vi "Scratch Module Selection.vi"(8 "error in (no error)":errorcluster, 11 "Data Cluster":T1) -> (0 "error out":errorcluster)   [LabVIEW 2025]
uses:
  controls/LAB-IQ UI Data.ctl
  Traction Loop/Traction Receipe Enum.ctl
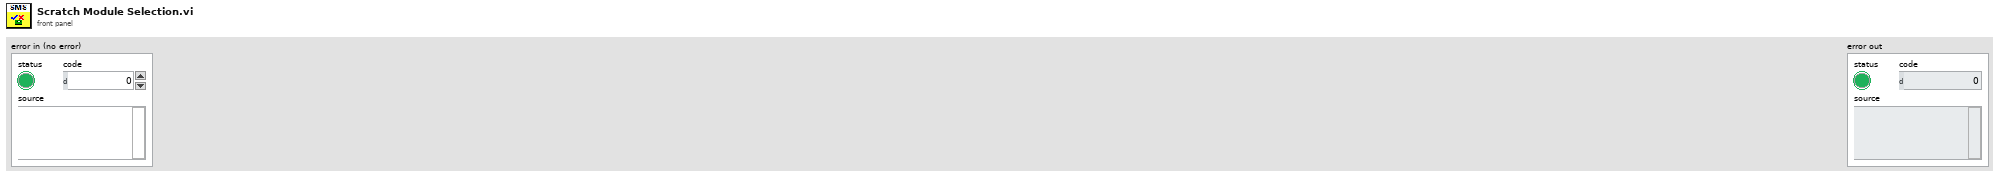
[diagram p1: front panel]
types:
  T1 = typedef "LAB-IQ UI Data.ctl" = cluster{"Main Home Screen":cluster{"GUI":refnum<vi>, "Platform Settings":refnum<vi>, "Configure":refnum<vi>, "Home":refnum<vi>, "EXIT":refnum<vi>, "service 2":refnum<vi>, "MainPage":refnum<vi>, "Analysis":refnum<vi>}, "Platform Settings":cluster{"mm/s  Surge":refnum<vi>, "Update Surge Speed":refnum<vi>, "Drive Error":refnum<vi>, "Disable Axis Jog Soft Limits":refnum<vi>, "mm/s  Sway":refnum<vi>, "Sway and Surge COM Status":refnum<vi>, "Heave COM Status":refnum<vi>, "Enable Platform":refnum<vi>, "Surge Forward Main":refnum<vi>, "Sway Right Main":refnum<vi>, "Sway Left Main":refnum<vi>, "Heave Down Main":refnum<vi>, "Heave Up main":refnum<vi>, "Update Sway Speed":refnum<vi>, "Update Heave Speed":refnum<vi>, "mm/s Heave":refnum<vi>, "mm/sec":refnum<vi>, "mm":refnum<vi>, "Surge Backward Main":refnum<vi>}, "Analysis Screen":cluster{"Analysis Home":refnum<vi>, "Surface Analysis":refnum<vi>, "Imaging":refnum<vi>, "Image Analysis":refnum<vi>, "Post Analysis":refnum<vi>}, "Config Screen":cluster{"Select Load Head":refnum<vi>, "Notes :":refnum<vi>, "FILE":refnum<vi>, "Sample ID :":refnum<vi>, "Operator ID :":refnum<vi>, "Operator Name :":refnum<vi>, "Auto":refnum<vi>}, "Motion Module":cluster{"zNL":refnum<vi>, "NL disp":refnum<vi>, "Rotary Tab":refnum<vi>, "Motion Direction:  3":refnum<vi>, "E.Velocity 2":refnum<vi>, "e.v/ssr 2":refnum<vi>, "Enter Fixed E.Velocity 2":refnum<vi>, "Enter Final SRR 2":refnum<vi>, "Enter initial SRR 2":refnum<vi>, "Enter Fixed SRR 2":refnum<vi>, "Enter the Final E.Velocity (m/s) 2":refnum<vi>, "Enter initial E.Velocity (m/s) 2":refnum<vi>, "Final Speed (RPM) 3":refnum<vi>, "Initial Speed (RPM) 2":refnum<vi>, "Enter the Final Velocity (m/s) 3":refnum<vi>, "Enter initial Velocity (m/s)  3":refnum<vi>, "Ramp Up 2":refnum<vi>, "TEST SELECTION":refnum<vi>, "SPEED SELECTION : ":refnum<vi>, "Angular Oscillation Set":refnum<vi>, "Traction":refnum<vi>, "Step Speed":refnum<vi>, "StepTable For Load-Speed":refnum<vi>, "StepTable For Speed":refnum<vi>, "Surge Forward MM":refnum<vi>, "Surge Backward MM":refnum<vi>, "M3 Image":refnum<vi>, "String 39":refnum<vi>, "Sway Left MM":refnum<vi>, "Sway Right MM":refnum<vi>, "Disable Axis Jog Soft Limits":refnum<vi>, "mm":refnum<vi>, "Heave Down MM":refnum<vi>, "Heave Up MM":refnum<vi>, "Wear Track Diameter (mm)":refnum<vi>, "Set WTD":refnum<vi>, "HomeScratch":refnum<vi>, "HomeRot":refnum<vi>, "PlaceModule":refnum<vi>, "Enter the Angle (Deg)":refnum<vi>, "Enter the Frequency (Hz)":refnum<vi>, "Motion Mode:":refnum<vi>, "LR Sway":refnum<vi>, "Rot Hor":refnum<vi>, "Scratch":refnum<vi>, "LR Cam":refnum<vi>, "MMBack":refnum<vi>, "MMNext":refnum<vi>, "Rot Ver":refnum<vi>, "Rotary Module Selection":refnum<vi>, "calculate rotary":refnum<vi>, "SPEED SELECTION : rotary":refnum<vi>, "Import 2":refnum<vi>, "Save 2":refnum<vi>, "File Path :  2":refnum<vi>, "String 45":refnum<vi>, "StepTable For Speed 3":refnum<vi>, "Enter the Speed(mm/sec)":refnum<vi>, "Enter the Speed(RPM)":refnum<vi>, "Enter Scratch Speed (mm/s):":refnum<vi>, "SwaySpeed Set":refnum<vi>, "Scartch Offset":refnum<vi>, "Motion type:":refnum<vi>, "HomeScratch 2":refnum<vi>, "Enter Scratch length (mm):":refnum<vi>, "Wear Track Diameter":refnum<vi>, "Rotary Speed Exced":refnum<vi>, "Scratch Mode":refnum<vi>, "No of Scratch":refnum<vi>}, "Environmental control":cluster{"Humidity  Status  3":refnum<vi>, "Low Temp  Status  2":refnum<vi>, "TK4 status 2":refnum<vi>, "Stage Temperature":refnum<vi>, "Sample Temperature":refnum<vi>, "Humidity (Amb)":refnum<vi>, "Clear List":refnum<vi>, "Add to list":refnum<vi>, "Wear":refnum<vi>, "Vibration":refnum<vi>, "Humidity (Chamber)":refnum<vi>, "Temperature (Chamber)":refnum<vi>, "ECR ":refnum<vi>, "Temperature (Amb)":refnum<vi>, "Microphone":refnum<vi>, "Acoustic Emission 3":refnum<vi>, "SNext":refnum<vi>, "APBack":refnum<vi>, "Enter the Temperature (°C):":refnum<vi>, "Enter the Stage \nTemperature (°C):":refnum<vi>, "Enter the Humidity (%Rh):":refnum<vi>, "Low Temp":refnum<vi>, "High Temp":refnum<vi>, "Humidity":refnum<vi>, "Sensors Picked":refnum<vi>}, "About Screen":cluster{"Password":refnum<vi>, "Home Service":refnum<vi>, "Advanced Setting":refnum<vi>, "About Tab":refnum<vi>, "ECR Port:":refnum<vi>, "Ramp Port:":refnum<vi>, "Installation/Replacement completed":refnum<vi>, "Loahead":refnum<vi>, "Heave and Surge COM Port:":refnum<vi>, "Sway COM Port:":refnum<vi>, "Temp Modbus:":refnum<vi>, "Humidity Port:":refnum<vi>, "Edit Gain Constants":refnum<vi>, "Save Gain Constants":refnum<vi>}, "Main Screen":cluster{"Main Screen Tab":refnum<vi>, "Angle and Frequency":refnum<vi>, "Stroke (mm)":refnum<vi>, "Angle (Deg)":refnum<vi>, "Main Speed Tab":refnum<vi>, "MTM MOTOR DISPLAY":refnum<vi>, "Disc Speed (m/sec)":refnum<vi>, "Ball Speed (m/sec)":refnum<vi>, "Disc Speed (RPM)":refnum<vi>, "Ball Speed (RPM)":refnum<vi>, "SPEED TAB":refnum<vi>, "Speed (m/sec)":refnum<vi>, "Set Speed (m/sec)":refnum<vi>, "Speed (RPM)":refnum<vi>, "Set Speed":refnum<vi>, "Time Tab":refnum<vi>, "Time ( HH:MM:SS ) 2":refnum<vi>, "Test Duration":refnum<vi>, "Test Duration 4":refnum<vi>, "TEST CYCLE":refnum<vi>, "TOTAL CYCLES":refnum<vi>, "Set Load (N)":refnum<vi>, "Temp Tabs":refnum<vi>, "Heater":refnum<vi>, "TK4 status":refnum<vi>, "ChamberTemp":refnum<vi>, "SetTmp":refnum<vi>, "Controller  Status":refnum<vi>, "ChamberTemp 2":refnum<vi>, "SetTmp 2":refnum<vi>, "Controller  Status 2":refnum<vi>, "ChamberTemp 3":refnum<vi>, "SetTmp 3":refnum<vi>, "Cooling":refnum<vi>, "Load Communication":refnum<vi>, "Ambient \nTemperature":refnum<vi>, "HumCOMStatus":refnum<vi>, "Ambient\n Humidity":refnum<vi>, "Freq (Hz)":refnum<vi>, "Load En":refnum<vi>, "NLt":refnum<vi>, "zNL 2":refnum<vi>, "Humidity On":refnum<vi>, "humidity disp":refnum<vi>, "Set Humidity":refnum<vi>, "NL disp 2":refnum<vi>, "Humidity On 2":refnum<vi>, "humidity disp 2":refnum<vi>, "Set Humidity 2":refnum<vi>, "NL disp 3":refnum<vi>, "AppLoadSeq scratch":refnum<vi>, "Stop Scratch":refnum<vi>, "ClrLog":refnum<vi>, "Trip Log":refnum<vi>, "STOP":refnum<vi>, "Start Test":refnum<vi>, "Test status":refnum<vi>, "AR Led":refnum<vi>, "Data":refnum<vi>, "Health":refnum<vi>, "Sway COM Status":refnum<vi>, "Heave COM Status":refnum<vi>, "Grp Tab":refnum<vi>, "Sub Graph":refnum<vi>, "SD (mm)":refnum<vi>, "Siliding distance Reset Graph":refnum<vi>, "SDGp":refnum<vi>, "Humidity Reset Graph":refnum<vi>, "HumrGp":refnum<vi>, "Acoustic Emission (mV)":refnum<vi>, "Aqucostic Reset Graph":refnum<vi>, "gACQUOS":refnum<vi>, "ECR RESET":refnum<vi>, "ECR":refnum<vi>, "Temperature Reset":refnum<vi>, "Acoustic Emission (mV) 2":refnum<vi>, "Aqucostic Reset Graph 2":refnum<vi>, "gACQUOS 2":refnum<vi>, "ECR RESET 2":refnum<vi>, "ECR 2":refnum<vi>, "Temperature Reset 2":refnum<vi>, "Temperature (deg c)":refnum<vi>, "Speed Reset Graph":refnum<vi>, "Speed Tab":refnum<vi>, "MTM DISC  SPEED":refnum<vi>, "MTM BALL SPEED":refnum<vi>, "speed mm/sec":refnum<vi>, "Hymidity":refnum<vi>, "Humidity Disable trip":refnum<vi>, "CoF Trip  2":refnum<vi>, "Depth Trip":refnum<vi>, "Weart Deapth":refnum<vi>, "Depth Reset Graph":refnum<vi>, "Weart":refnum<vi>, "Depthz":refnum<vi>, "Depth (µm)":refnum<vi>, "WearGp":refnum<vi>, "NL Trip 2":refnum<vi>, "Load pid":refnum<vi>, "Load Disable Trip":refnum<vi>, "Load Reset Graph":refnum<vi>, "NL Display 4":refnum<vi>, "Main Chart 3":refnum<vi>, "BACK":refnum<vi>, "Depth Trip 2":refnum<vi>, "COF TRIP ":refnum<vi>, "Friction Force (N)":refnum<vi>, "FF Reset Graph":refnum<vi>, "FF Disable Trip":refnum<vi>, "FF TRIP":refnum<vi>, "COF Disable Trip":refnum<vi>, "COF Reset Graph":refnum<vi>, "Start Test Temp":refnum<vi>, "zFF":refnum<vi>, "Friction Force (N) Graph":refnum<vi>, "Coefficient of Friction":refnum<vi>, "Scratch Start Test":refnum<vi>, "FF Tab":refnum<vi>, "Cyclic Friction Force (N)":refnum<vi>, "CZ FF":refnum<vi>, "Cyclic Friction Force (N) Graph":refnum<vi>, "Cyclic Coefficient of Friction":refnum<vi>, "Cyclic FF TRIP":refnum<vi>, "Cyclic FF Disable Trip":refnum<vi>, "cyclic COF Disable Trip":refnum<vi>, "cyclic COF TRIP":refnum<vi>, "cyclic COF Reset Graph":refnum<vi>, "Cyclic FF Reset Graph":refnum<vi>, "Test Trip":refnum<vi>, "Multi Scratch Pass":refnum<vi>, "Scratch Start Recording":refnum<vi>}, "Loading":cluster{"Indentation":refnum<vi>, "Reference Sample":refnum<vi>, "Load Cell Communication Slide":refnum<vi>, "com 3":refnum<vi>, "com":refnum<vi>, "DecaForce COM Status":refnum<vi>, "Update":refnum<vi>, "Clear 3":refnum<vi>, "seq":refnum<vi>, "Stribeck table":refnum<vi>, "Stribeck Table  For loading":refnum<vi>, "Loading Mode":refnum<vi>, "Enter the Final Load (N)":refnum<vi>, "Enter the CoF Trip":refnum<vi>, "Enter the Friction Force Trip":refnum<vi>, "Enter the Normal load Trip":refnum<vi>, "Enter the Load  (N)":refnum<vi>, "KiloForce":refnum<vi>, "DecaForce ":refnum<vi>, "MicroForce":refnum<vi>, "LHBack":refnum<vi>, "LHNext":refnum<vi>, "Enter the Loading Rate (N/min)":refnum<vi>, "Message":refnum<vi>, "Warning 2":refnum<vi>, "SSP 0.75":refnum<vi>, "SSP 0.5":refnum<vi>, "SSP 0.3":refnum<vi>, "Warning":refnum<vi>, "gui GIF":refnum<vi>, "Communication is established":refnum<vi>, "AppLoad 4":refnum<vi>, "Multipoint":refnum<vi>, "Load Selection":refnum<vi>}, "PID":cluster{"Ramp MulFac":refnum<vi>, "pulses LoadDiffRamp(2..10)":refnum<vi>, "PulseControlRamp(diff<=3N)":refnum<vi>, "SetLoadDeadband(%) Load(0-10N)":refnum<vi>, "PID gains out delay (microForce)":refnum<vi>, "Ramp":refnum<vi>, "Gain 2":refnum<vi>, "pulses LoadDiff(2..10)":refnum<vi>, "pulses LoadDiff(11..50)":refnum<vi>, "PulseControl(diff<=3N)":refnum<vi>, "SetLoadDeadband(%)  2":refnum<vi>, "Dummy Run":refnum<vi>, "Vertical load (N)":refnum<vi>, "AutoTune":refnum<vi>, "Offset 3 ":refnum<vi>, "apply load":refnum<vi>, "Offset  3":refnum<vi>, "apply load 2":refnum<vi>, "Enter ByPass Load":refnum<vi>, "reinit 3":refnum<vi>, "output range delay":refnum<vi>, "PID gains out delay":refnum<vi>, "Bypass Load":refnum<vi>, "pulsesSent":refnum<vi>, "pulses ":refnum<vi>, "actpid":refnum<vi>, "gFF Rot":refnum<vi>, "pulses LoadDiff(21..1000)":refnum<vi>, "Delay":refnum<vi>, "deadband":refnum<vi>}, "Config Parameters":cluster{"Tab Control 3":refnum<vi>, "Tab Control 19":refnum<vi>, "SAMPLES":refnum<vi>, "Re-initilaize":refnum<vi>, "Filter ON/OFF":refnum<vi>, "TracHomeSurgeOffsetCounts 10MM":refnum<vi>, "TracHomeSwayOffsetCounts 10MM":refnum<vi>, "Acoustic Emission:":refnum<vi>, "Apply Filter (FF)":refnum<vi>, "Filter% 2":refnum<vi>, "Apply Filter (Load)":refnum<vi>, "Filter% ":refnum<vi>, "Sway distance (mm)":refnum<vi>, "Surge distance (mm)":refnum<vi>, "DataSavingLoopDelay(ms)":refnum<vi>, "SAVE 2":refnum<vi>, "Enter Distance":refnum<vi>, "Sway Counts:":refnum<vi>, "Distance (mm): 3":refnum<vi>, "Surge Counts:":refnum<vi>, "Distance (mm): 2":refnum<vi>, "Distance (mm):":refnum<vi>, "Heave Counts:":refnum<vi>, "LRMHomeSurgeOffsetCounts":refnum<vi>, "LRMHomeSwayOffsetCounts":refnum<vi>, "TracHomeSurgeOffsetCounts 20MM":refnum<vi>, "TracHomeSwayOffsetCounts 20MM":refnum<vi>, "RotHomeSwayOffsetCounts":refnum<vi>, "RotHomeSurgeOffsetCounts":refnum<vi>, "Heave distance":refnum<vi>, "Zmm":refnum<vi>, "Heave Pulses/mm":refnum<vi>, "Surge Pulses/mm":refnum<vi>, "Sway Pulses/mm":refnum<vi>, "Heave Pitch":refnum<vi>, "Surge Pitch":refnum<vi>, "Sway Pitch":refnum<vi>, "Heave PPR":refnum<vi>, "Surge PPR":refnum<vi>, "Sway PPR":refnum<vi>, "Tab Control 5":refnum<vi>, "Tab Control 14":refnum<vi>, "Tab Control 26":refnum<vi>, "AE":refnum<vi>, "Heave Loop Delay":refnum<vi>, "Heave PID Speed":refnum<vi>, "Surge Jog Speed":refnum<vi>, "Heave Jog Speed":refnum<vi>, "Sway Loop Delay":refnum<vi>, "Sway PID Speed":refnum<vi>, "Sway Jog Speed":refnum<vi>, "DEPTH TRIP VALUE":refnum<vi>, "LOAD TRIP VALUE":refnum<vi>, "DEPTH TRIP   ENABLE":refnum<vi>, "LOAD TRIP  ENABLE":refnum<vi>, "CYCLIC FF TRIP VALUE":refnum<vi>, "FF TRIP VALUE":refnum<vi>, "CYCLIC CoF TRIP VALUE":refnum<vi>, "COF TRIP VALUE":refnum<vi>, "CYCLIC COF TRIP  ENABLE":refnum<vi>, "CYCLIC FF TRIP  ENABLE":refnum<vi>, "FF TRIP  ENABLE":refnum<vi>, "COF TRIP  ENABLE":refnum<vi>, "JOG TRIP LOAD VALUE (N)":refnum<vi>}, "Loading Com Port":cluster{"ClearAll":refnum<vi>, "Mz(Nm)":refnum<vi>, "My(Nm)":refnum<vi>, "Mx(Nm)":refnum<vi>, "Save Dwell":refnum<vi>, "Mx ":refnum<vi>, "My ":refnum<vi>, "Mz":refnum<vi>, "Fx(N)":refnum<vi>, "Fy(N)":refnum<vi>, "Fz(N)":refnum<vi>, "ZeroAll":refnum<vi>, "Acq Delay (ms)":refnum<vi>, "Burst Delay (ms)":refnum<vi>, "model":refnum<vi>, "SN":refnum<vi>, "FFx(N)":refnum<vi>, "Sensor IP":refnum<vi>, "Port":refnum<vi>, "FFy(N)":refnum<vi>, "Load(N)":refnum<vi>, "delete Handle":refnum<vi>, "Create Handle":refnum<vi>, "ft_data":refnum<vi>, "ft_range":refnum<vi>, "ft_data 2":refnum<vi>, "stop 6":refnum<vi>, "running_flag":refnum<vi>, "ft_udp_handle":refnum<vi>, "get-data-return":refnum<vi>, "get-range-return":refnum<vi>, "zero-return":refnum<vi>, "filter-return":refnum<vi>, "initial-return":refnum<vi>, "deleteHandle-result":refnum<vi>, "Load Cell Temp":refnum<vi>}, "Heave AND Surge":cluster{"SURGE POSE":refnum<vi>, "error out Read":refnum<vi>, "HEAVE POSE":refnum<vi>, "State":refnum<vi>, "Homed":refnum<vi>, "Sequence ID":refnum<vi>, "error out Write":refnum<vi>, "faultCode":refnum<vi>, "Ack ID":refnum<vi>, "SPEED":refnum<vi>, "Distance":refnum<vi>, "Mode Command":refnum<vi>, "Heave and Surge Read":refnum<vi>, "Read Heave Temp":refnum<vi>, "Spare 15":refnum<vi>, "Spare 14":refnum<vi>, "Spare 13":refnum<vi>, "Spare 12":refnum<vi>, "Spare 11":refnum<vi>, "Spare 10":refnum<vi>, "Spare 9":refnum<vi>, "Spare 8":refnum<vi>, "Spare 7":refnum<vi>, "Spare 6":refnum<vi>, "Spare 5":refnum<vi>, "Spare 4":refnum<vi>, "Spare 2":refnum<vi>, "Spare 1":refnum<vi>, "Node Id":refnum<vi>, "Spare 3":refnum<vi>, "SPARE 4":refnum<vi>, "SPARE 3":refnum<vi>, "SPARE 2":refnum<vi>, "SPARE 1":refnum<vi>, "fwMajor":refnum<vi>, "fwMinor":refnum<vi>, "Manual Write":refnum<vi>, "Heave and Surge Write":refnum<vi>, "SPARE 5":refnum<vi>, "Reserved ":refnum<vi>, "SPARE 8":refnum<vi>, "SPARE 6":refnum<vi>, "SPARE 7":refnum<vi>, "SPARE 17":refnum<vi>, "SPARE 16":refnum<vi>, "SPARE 15":refnum<vi>, "SPARE 14":refnum<vi>, "SPARE 13":refnum<vi>, "SPARE 12":refnum<vi>, "SPARE 11":refnum<vi>, "SPARE 10":refnum<vi>, "SPARE 9":refnum<vi>, "System UPTIME":refnum<vi>, "Missed Packets":refnum<vi>, "faultCode Surge Right":refnum<vi>, "faultCode Surge Left":refnum<vi>, "faultCode Heave":refnum<vi>}, "New PID LOGIC":cluster{"Fine Tune Zone":refnum<vi>, "PID SDelay":refnum<vi>, "Max_pos_limit":refnum<vi>, "Min_pos_limit":refnum<vi>, "i_limit":refnum<vi>, "pct_scale":refnum<vi>, "Deadband":refnum<vi>, "Kd":refnum<vi>, "Ki":refnum<vi>, "Kp":refnum<vi>, "Current Position":refnum<vi>, "Set Load":refnum<vi>, "Current Load":refnum<vi>, "Pulse delta":refnum<vi>, "Init Step":refnum<vi>, "Max Step Linit":refnum<vi>, "min_deadband_floor":refnum<vi>, "dynamic_spindle_noise_scalar":refnum<vi>, "min_finetune_floor":refnum<vi>, "filter_alpha":refnum<vi>}, "SWAY ":cluster{"fwMajor":refnum<vi>, "Homed":refnum<vi>, "Rotary POSE":refnum<vi>, "State":refnum<vi>, "SWAY POSE":refnum<vi>, "Ack ID":refnum<vi>, "faultCode":refnum<vi>, "Node Id":refnum<vi>, "fwMinor":refnum<vi>, "Spare 6":refnum<vi>, "Spare 5":refnum<vi>, "Spare 4":refnum<vi>, "Spare 3":refnum<vi>, "Spare 2":refnum<vi>, "Spare 1":refnum<vi>, "Spare 7":refnum<vi>, "SPARE  5":refnum<vi>, "error out Write  SWAY ":refnum<vi>, "error out Read SWAY ":refnum<vi>, "Manual Write SWAY ":refnum<vi>, "SWAY WRITE":refnum<vi>, "SPARE  4":refnum<vi>, "SPARE  3":refnum<vi>, "SPARE 2":refnum<vi>, "SPARE 1":refnum<vi>, "Spare 15":refnum<vi>, "Spare 14":refnum<vi>, "Spare 13":refnum<vi>, "Spare 12":refnum<vi>, "Spare 11":refnum<vi>, "Spare 9":refnum<vi>, "Spare 8":refnum<vi>, "SPEED":refnum<vi>, "Distance":refnum<vi>, "Mode Command":refnum<vi>, "Sequence ID":refnum<vi>, "SWAY READ":refnum<vi>, "Spare 10":refnum<vi>, "Read SWAY Temp":refnum<vi>, "faultCode Sway ":refnum<vi>, "Missed Packets":refnum<vi>, "System UPTIME sway":refnum<vi>, "SPARE 6":refnum<vi>, "SPARE 7":refnum<vi>, "SPARE 9":refnum<vi>, "SPARE 11":refnum<vi>, "SPARE 10":refnum<vi>, "SPARE 8":refnum<vi>, "SPARE 13":refnum<vi>, "SPARE 12":refnum<vi>, "SPARE 17":refnum<vi>, "SPARE 16":refnum<vi>, "SPARE 15":refnum<vi>, "SPARE 14":refnum<vi>, "Reserved":refnum<vi>, "faultCode Rotary":refnum<vi>}, "Analysis Screen":cluster{"Analysis Home":refnum<vi>, "Refresh 2":refnum<vi>, "MEAN 4":refnum<vi>, "SD 4":refnum<vi>, "VARIANCE 4":refnum<vi>, "MEAN  3":refnum<vi>, "SD  3":refnum<vi>, "VARIANCE  3":refnum<vi>, "MEAN 2":refnum<vi>, "SD  2":refnum<vi>, "VARIANCE 2":refnum<vi>, "MEAN":refnum<vi>, "SD":refnum<vi>, "VARIANCE":refnum<vi>, "File 4 Discription":refnum<vi>, "OPEN 4":refnum<vi>, "File Name 4":refnum<vi>, "OPEN 3":refnum<vi>, "File 3 Discription":refnum<vi>, "File Name 3":refnum<vi>, "Y-AXIS":refnum<vi>, "X-AXIS":refnum<vi>, "XY Graph":refnum<vi>, "File Name 2":refnum<vi>, "File Name 1":refnum<vi>, "OPEN 2":refnum<vi>, "OPEN 1":refnum<vi>, "File 1 Discription ":refnum<vi>, "File 2 Discription":refnum<vi>, "Export":refnum<vi>, "File Format":refnum<vi>}, "Traction":cluster{"faultCode Traction 2":refnum<vi>, "faultCode Traction 1":refnum<vi>, "Missed Packets":refnum<vi>, "System UPTIME Traction":refnum<vi>, "SPARE 17":refnum<vi>, "SPARE 16":refnum<vi>, "SPARE 15":refnum<vi>, "SPARE 14":refnum<vi>, "SPARE 13":refnum<vi>, "SPARE 12":refnum<vi>, "SPARE 11":refnum<vi>, "SPARE 10":refnum<vi>, "SPARE 9":refnum<vi>, "SPARE 8":refnum<vi>, "SPARE 7":refnum<vi>, "SPARE 6":refnum<vi>, "Reserved":refnum<vi>, "SPARE  5":refnum<vi>, "Manual Write TRACTION":refnum<vi>, "TRACTION WRITE":refnum<vi>, "SPARE  4":refnum<vi>, "SPARE  3":refnum<vi>, "SPARE 2":refnum<vi>, "SPARE 1":refnum<vi>, "Spare 7":refnum<vi>, "Spare 6":refnum<vi>, "Spare 5":refnum<vi>, "Spare 4":refnum<vi>, "Spare 2":refnum<vi>, "Spare 1":refnum<vi>, "Node Id":refnum<vi>, "Read TRACTION Temp":refnum<vi>, "fwMinor":refnum<vi>, "fwMajor":refnum<vi>, "faultCode":refnum<vi>, "TRACTION POSE":refnum<vi>, "TRACTION POSE 2":refnum<vi>, "Homed":refnum<vi>, "State":refnum<vi>, "Ack ID":refnum<vi>, "SPEED":refnum<vi>, "Distance":refnum<vi>, "Mode Command":refnum<vi>, "Sequence ID":refnum<vi>, "error out Read TRACTION":refnum<vi>, "error out Write  TRACTION":refnum<vi>, "TRACTION READ":refnum<vi>, "Spare 3":refnum<vi>}, "Traction reciepe":cluster{"SRR Sweep Range (%) Stribeck":refnum<vi>, "Traction Receipe":refnum<vi>, "Total Execution Time":refnum<vi>, "Total Steps":refnum<vi>, "Duration / Step (s)  Stribeck":refnum<vi>, "STRIBECK Fixed SRR List (%)":refnum<vi>, "Duration / Step (s) Traction":refnum<vi>, "SRR Sweep Range (%) traction":refnum<vi>, "Rolling Speed (mm/s)":refnum<vi>, "Temperature Stages (°C)":refnum<vi>, "Ball Load (N)":refnum<vi>, "Lubricant Name":refnum<vi>, "Profile File Name":refnum<vi>, "SET entrainment Velocity":refnum<vi>, "Test Array Size":refnum<vi>, "SRR INDEX [ STRIBECK]":refnum<vi>, "Stribeck Size":refnum<vi>, "SET SRR":refnum<vi>, "ELAPSED TIMER ":refnum<vi>, "BALL SET RPM":refnum<vi>, "DISC SET RPM":refnum<vi>, "SET LOAD":refnum<vi>, "TEMPERATURE READ":refnum<vi>, "SET TEMPERATURE":refnum<vi>, "Traction Size":refnum<vi>, "DISC SPEED (rpm)":refnum<vi>, "BALL SPEED (rpm)":refnum<vi>, "BALL WEAR TRACK":refnum<vi>, "DISC WEARTRACK":refnum<vi>, "SRR INDEX [ TRACTION]":refnum<vi>, "Start Index Type":refnum<vi>, "Enum - Menu":refnum<vi>, "Ball (mm/sec)":refnum<vi>, "Disc (mm/sec)":refnum<vi>}, "Traction Control":cluster{"HomeTraction":refnum<vi>, "Demo Mode Display":refnum<vi>, "Traction Message":refnum<vi>, "Traction Step Update Details":refnum<vi>, "Main Tab sequence for selection":refnum<vi>, "Ramp Tab":refnum<vi>, "e.v/ssr":refnum<vi>, "Enter Fixed E.Velocity":refnum<vi>, "Enter Final SRR":refnum<vi>, "Enter initial SRR":refnum<vi>, "Enter Fixed SRR":refnum<vi>, "Enter the Final E.Velocity (m/s)":refnum<vi>, "Enter initial E.Velocity (m/s)":refnum<vi>, "Ball WTD":refnum<vi>, "E.Velocity":refnum<vi>, "Enter the Final Velocity (m/s)":refnum<vi>, "Enter initial Velocity (m/s)":refnum<vi>, "Ramp Up   Disc":refnum<vi>, "Initial DiscSpeed (RPM)":refnum<vi>, "Final Speed (RPM) Ball":refnum<vi>, "Final Speed (RPM)":refnum<vi>, "Initial Speed (RPM) Ball":refnum<vi>, "Enter the Final Velocity (m/s) Ball":refnum<vi>, "Enter initial Velocity (m/s) Ball":refnum<vi>, "Ramp Up":refnum<vi>, "ExceedBallSpeed step":refnum<vi>, "ExceedDiscSpeed":refnum<vi>, "BallSpeed Exceed Indication":refnum<vi>, "Apply":refnum<vi>, "SPEED SELECTION : MTM":refnum<vi>, "SPEED SELECTION : MTM 2":refnum<vi>, "TEST SELECTION (MTM)":refnum<vi>, "MTM Test Selection":refnum<vi>, "File Path Tab":refnum<vi>, "File Path String":refnum<vi>, "Save":refnum<vi>, "Save  2":refnum<vi>, "Import ":refnum<vi>, "File Path :":refnum<vi>, "Step Sequence Indication Tab":refnum<vi>, "Step Sequence Indication":refnum<vi>, "Calculate Step":refnum<vi>, "StepTable":refnum<vi>, "ExceedDiscSpeed  Cinstant Speed":refnum<vi>, "ExceedBallSpeed Constant":refnum<vi>, "TEST SELECTION (MTM) 2":refnum<vi>, "SPEED SELECTION : MTM 3":refnum<vi>, "MTM Test Selection 2":refnum<vi>, "Enter the Speed (m/sec): ":refnum<vi>, "Enter the Speed (m/sec):  2":refnum<vi>, "Enter the Speed (RPM):":refnum<vi>, "Lower Spped ":refnum<vi>, "Upper":refnum<vi>, "Enter the Speed (RPM):Ball":refnum<vi>, "Disc Motion Direction: ":refnum<vi>, "Ball Motion Direction :":refnum<vi>, "Motion Mode: ":refnum<vi>, "Wear Track Diameter (mm) ":refnum<vi>, "Disc Speed Indicator":refnum<vi>, "ExceedBallSpeed":refnum<vi>}, "Acquostic":cluster{"Last Config Rejected ":refnum<vi>, "rx command count":refnum<vi>, "Current Filter Id":refnum<vi>, "Isolated Gain":refnum<vi>, "DAQ Status":refnum<vi>, "error out":refnum<vi>, "error in (no error)":refnum<vi>, "Uplink Packet":refnum<vi>, "data out":refnum<vi>, "Downlink Packet":refnum<vi>, "Signal Energy":refnum<vi>, "Amplitude db_AE":refnum<vi>, "Peak Amplitude":refnum<vi>, "AE Ring-Down Counts":refnum<vi>, "Gains":refnum<vi>, "Manual Write Acquostic":refnum<vi>}}
  T2 = enum32{"Details", "PlatformSetting", "Analysis", "HOME"}
  T3 = enum32{"Setup", "Load Head", "Motion Module", "Environment", "Begin"}
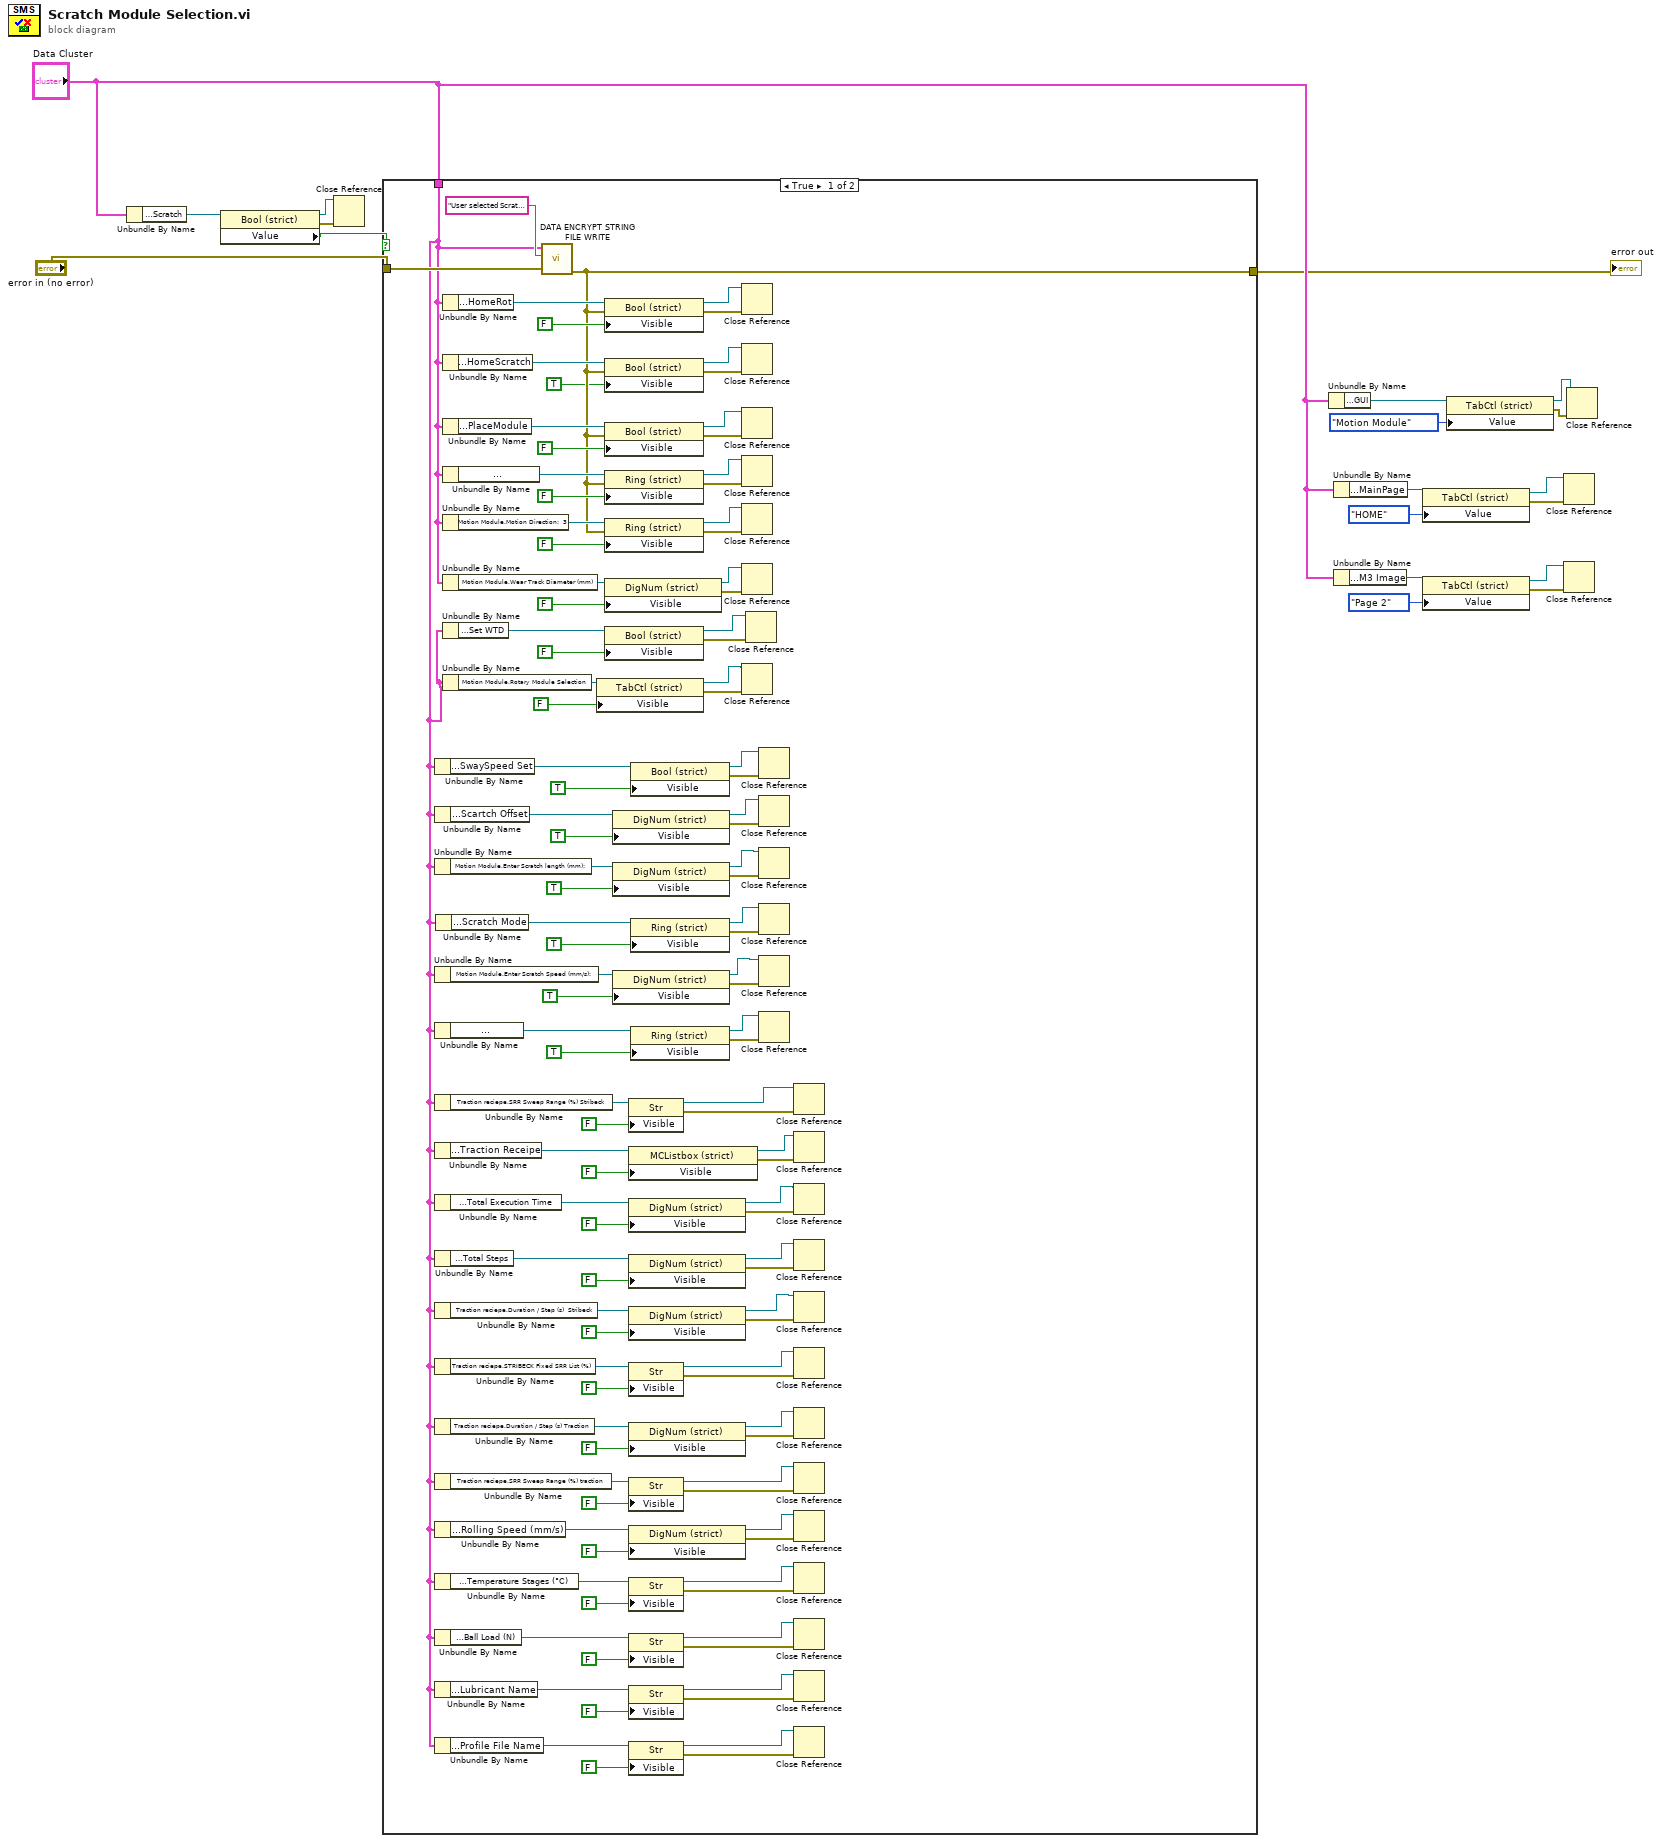
[diagram p0: block diagram]
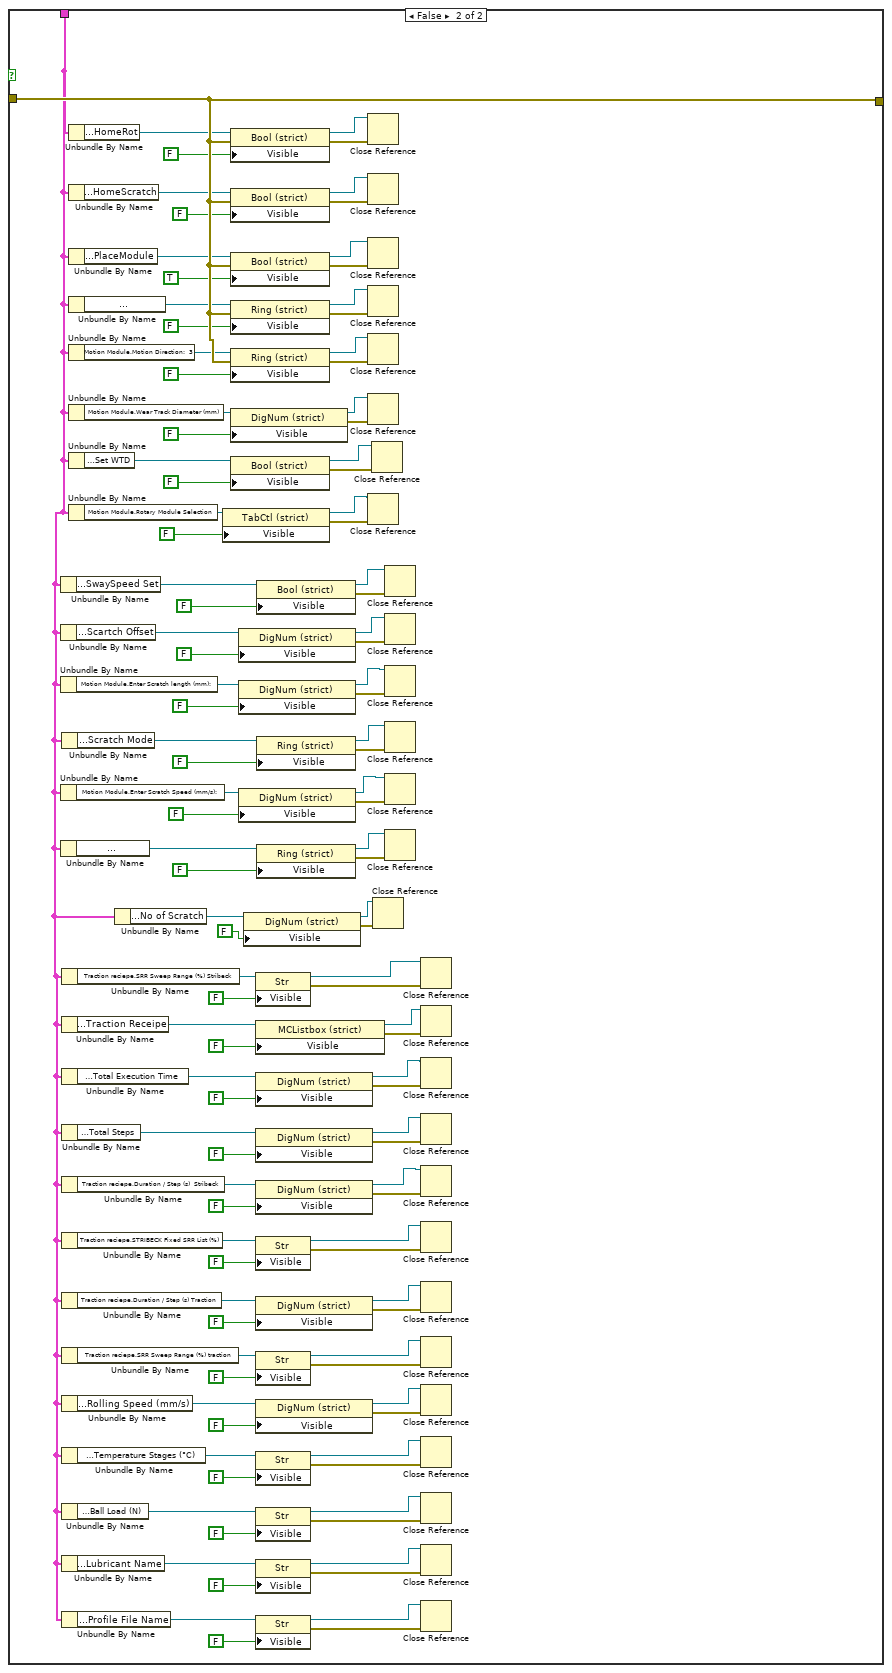
[diagram p2: hidden frame]
diagram:
  n1 = Unbundle By Name("Data Cluster") -> ("Motion Module.Scratch"=w17:refnum<vi>)
  n2 = property class="Bool (strict)"(reference=w17) -> (reference out=w15:refnum<vi>, error out=w16:errorcluster, "Value"=w19:bool)  [unwired: 1 in]
  n3 = Close Reference(reference=w15, error in (no error)=w16) -> ()  [unwired: 1 out]
  n4 = case shown="True" w19 {
    tunnel: "error in (no error)" -> [w130 w245]
    tunnel: [w102 w245] -> w10
    tunnel: "Data Cluster" -> [w20 w132]
    frame True {
      n5 = Unbundle By Name(w20) -> ("Motion Module.SwaySpeed Set"=w89:refnum<vi>)
      n6 = Unbundle By Name(w20) -> ("Motion Module.Scartch Offset"=w92:refnum<vi>)
      n7 = Unbundle By Name(w20) -> ("Motion Module.Enter Scratch length (mm):"=w95:refnum<vi>)
      n8 = Unbundle By Name(w20) -> ("Motion Module.Enter Scratch Speed (mm/s):"=w84:refnum<vi>)
      n9 = Unbundle By Name(w20) -> ("Motion Module.Motion type:"=w81:refnum<vi>)
      n10 = Unbundle By Name(w20) -> ("Traction reciepe.SRR Sweep Range (%) Stribeck"=w55:refnum<vi>)
      n11 = Unbundle By Name(w20) -> ("Traction reciepe.Traction Receipe"=w58:refnum<vi>)
      n12 = Unbundle By Name(w20) -> ("Traction reciepe.Total Execution Time"=w61:refnum<vi>)
      n13 = Unbundle By Name(w20) -> ("Traction reciepe.Total Steps"=w53:refnum<vi>)
      n14 = Unbundle By Name(w20) -> ("Traction reciepe.Duration / Step (s)  Stribeck"=w50:refnum<vi>)
      n15 = Unbundle By Name(w20) -> ("Traction reciepe.STRIBECK Fixed SRR List (%)"=w47:refnum<vi>)
      n16 = Unbundle By Name(w20) -> ("Traction reciepe.Duration / Step (s) Traction"=w70:refnum<vi>)
      n17 = Unbundle By Name(w20) -> ("Traction reciepe.SRR Sweep Range (%) traction"=w34:refnum<vi>)
      n18 = Unbundle By Name(w20) -> ("Traction reciepe.Rolling Speed (mm/s)"=w31:refnum<vi>)
      n19 = Unbundle By Name(w20) -> ("Traction reciepe.Temperature Stages (°C)"=w28:refnum<vi>)
      n20 = Unbundle By Name(w20) -> ("Traction reciepe.Ball Load (N)"=w36:refnum<vi>)
      n21 = Unbundle By Name(w20) -> ("Traction reciepe.Lubricant Name"=w39:refnum<vi>)
      n22 = Unbundle By Name(w20) -> ("Traction reciepe.Profile File Name"=w42:refnum<vi>)
      n23 = Unbundle By Name(w20) -> ("Motion Module.Scratch Mode"=w87:refnum<vi>)
      n24 = Unbundle By Name(w20) -> ("Motion Module.HomeRot"=w129:refnum<vi>)
      n25 = Unbundle By Name(w20) -> ("Motion Module.HomeScratch"=w124:refnum<vi>)
      n26 = Unbundle By Name(w20) -> ("Motion Module.PlaceModule"=w122:refnum<vi>)
      n27 = Unbundle By Name(w20) -> ("Motion Module.Motion Mode:"=w115:refnum<vi>)
      n28 = Unbundle By Name(w20) -> ("Motion Module.Motion Direction:  3"=w114:refnum<vi>)
      n29 = Unbundle By Name(w20) -> ("Motion Module.Wear Track Diameter (mm)"=w108:refnum<vi>)
      n30 = Unbundle By Name(w20) -> ("Motion Module.Set WTD"=w105:refnum<vi>)
      n31 = Unbundle By Name(w20) -> ("Motion Module.Rotary Module Selection"=w99:refnum<vi>)
      n32 = call "DATA ENCRYPT STRING FILE WRITE.vi"("error in (no error)"=w130, "User Action"="User selected Scratch Module", "main ref"=w20) -> ("error out"=w102:errorcluster)  [unwired: 6 in, 1 out]
      n33 = property class="TabCtl (strict)"(reference=w99, "Visible"=FALSE) -> (reference out=w98:refnum<vi>, error out=w100:errorcluster)  [unwired: 1 in]
      n34 = property class="Bool (strict)"(reference=w129, error in=w102, "Visible"=FALSE) -> (reference out=w127:refnum<vi>, error out=w128:errorcluster)
      n35 = property class="Bool (strict)"(reference=w124, error in=w102, "Visible"=TRUE) -> (reference out=w126:refnum<vi>, error out=w125:errorcluster)
      n36 = property class="Bool (strict)"(reference=w122, error in=w102, "Visible"=FALSE) -> (reference out=w120:refnum<vi>, error out=w121:errorcluster)
      n37 = property class="Ring (strict)"(reference=w115, error in=w102, "Visible"=FALSE) -> (reference out=w117:refnum<vi>, error out=w116:errorcluster)
      n38 = property class="Ring (strict)"(reference=w114, error in=w102, "Visible"=FALSE) -> (reference out=w111:refnum<vi>, error out=w113:errorcluster)
      n39 = property class="DigNum (strict)"(reference=w108, "Visible"=FALSE) -> (reference out=w107:refnum<vi>, error out=w109:errorcluster)  [unwired: 1 in]
      n40 = property class="Bool (strict)"(reference=w105, "Visible"=FALSE) -> (reference out=w106:refnum<vi>, error out=w104:errorcluster)  [unwired: 1 in]
      n41 = property class="DigNum (strict)"(reference=w92, "Visible"=TRUE) -> (reference out=w91:refnum<vi>, error out=w93:errorcluster)  [unwired: 1 in]
      n42 = property class="DigNum (strict)"(reference=w95, "Visible"=TRUE) -> (reference out=w96:refnum<vi>, error out=w94:errorcluster)  [unwired: 1 in]
      n43 = property class="DigNum (strict)"(reference=w84, "Visible"=TRUE) -> (reference out=w83:refnum<vi>, error out=w85:errorcluster)  [unwired: 1 in]
      n44 = property class="Str"(reference=w55, "Visible"=FALSE) -> (reference out=w56:refnum<vi>, error out=w54:errorcluster)  [unwired: 1 in]
      n45 = property class="MCListbox (strict)"(reference=w58, "Visible"=FALSE) -> (reference out=w57:refnum<vi>, error out=w59:errorcluster)  [unwired: 1 in]
      n46 = property class="DigNum (strict)"(reference=w61, "Visible"=FALSE) -> (reference out=w62:refnum<vi>, error out=w60:errorcluster)  [unwired: 1 in]
      n47 = property class="DigNum (strict)"(reference=w53, "Visible"=FALSE) -> (reference out=w48:refnum<vi>, error out=w52:errorcluster)  [unwired: 1 in]
      n48 = property class="DigNum (strict)"(reference=w50, "Visible"=FALSE) -> (reference out=w49:refnum<vi>, error out=w51:errorcluster)  [unwired: 1 in]
      n49 = property class="Str"(reference=w47, "Visible"=FALSE) -> (reference out=w45:refnum<vi>, error out=w46:errorcluster)  [unwired: 1 in]
      n50 = property class="DigNum (strict)"(reference=w70, "Visible"=FALSE) -> (reference out=w72:refnum<vi>, error out=w71:errorcluster)  [unwired: 1 in]
      n51 = property class="Str"(reference=w34, "Visible"=FALSE) -> (reference out=w33:refnum<vi>, error out=w35:errorcluster)  [unwired: 1 in]
      n52 = property class="DigNum (strict)"(reference=w31, "Visible"=FALSE) -> (reference out=w32:refnum<vi>, error out=w30:errorcluster)  [unwired: 1 in]
      n53 = property class="Str"(reference=w28, "Visible"=FALSE) -> (reference out=w27:refnum<vi>, error out=w29:errorcluster)  [unwired: 1 in]
      n54 = property class="Str"(reference=w36, "Visible"=FALSE) -> (reference out=w41:refnum<vi>, error out=w37:errorcluster)  [unwired: 1 in]
      n55 = property class="Str"(reference=w39, "Visible"=FALSE) -> (reference out=w40:refnum<vi>, error out=w38:errorcluster)  [unwired: 1 in]
      n56 = property class="Str"(reference=w42, "Visible"=FALSE) -> (reference out=w44:refnum<vi>, error out=w43:errorcluster)  [unwired: 1 in]
      n57 = property class="Bool (strict)"(reference=w89, "Visible"=TRUE) -> (reference out=w90:refnum<vi>, error out=w88:errorcluster)  [unwired: 1 in]
      n58 = property class="Ring (strict)"(reference=w87, "Visible"=TRUE) -> (reference out=w82:refnum<vi>, error out=w86:errorcluster)  [unwired: 1 in]
      n59 = property class="Ring (strict)"(reference=w81, "Visible"=TRUE) -> (reference out=w79:refnum<vi>, error out=w80:errorcluster)  [unwired: 1 in]
      n60 = Close Reference(reference=w127, error in (no error)=w128) -> ()  [unwired: 1 out]
      n61 = Close Reference(reference=w126, error in (no error)=w125) -> ()  [unwired: 1 out]
      n62 = Close Reference(reference=w120, error in (no error)=w121) -> ()  [unwired: 1 out]
      n63 = Close Reference(reference=w117, error in (no error)=w116) -> ()  [unwired: 1 out]
      n64 = Close Reference(reference=w111, error in (no error)=w113) -> ()  [unwired: 1 out]
      n65 = Close Reference(reference=w107, error in (no error)=w109) -> ()  [unwired: 1 out]
      n66 = Close Reference(reference=w98, error in (no error)=w100) -> ()  [unwired: 1 out]
      n67 = Close Reference(reference=w106, error in (no error)=w104) -> ()  [unwired: 1 out]
      n68 = Close Reference(reference=w90, error in (no error)=w88) -> ()  [unwired: 1 out]
      n69 = Close Reference(reference=w91, error in (no error)=w93) -> ()  [unwired: 1 out]
      n70 = Close Reference(reference=w96, error in (no error)=w94) -> ()  [unwired: 1 out]
      n71 = Close Reference(reference=w82, error in (no error)=w86) -> ()  [unwired: 1 out]
      n72 = Close Reference(reference=w83, error in (no error)=w85) -> ()  [unwired: 1 out]
      n73 = Close Reference(reference=w79, error in (no error)=w80) -> ()  [unwired: 1 out]
      n74 = Close Reference(reference=w56, error in (no error)=w54) -> ()  [unwired: 1 out]
      n75 = Close Reference(reference=w57, error in (no error)=w59) -> ()  [unwired: 1 out]
      n76 = Close Reference(reference=w62, error in (no error)=w60) -> ()  [unwired: 1 out]
      n77 = Close Reference(reference=w48, error in (no error)=w52) -> ()  [unwired: 1 out]
      n78 = Close Reference(reference=w49, error in (no error)=w51) -> ()  [unwired: 1 out]
      n79 = Close Reference(reference=w45, error in (no error)=w46) -> ()  [unwired: 1 out]
      n80 = Close Reference(reference=w72, error in (no error)=w71) -> ()  [unwired: 1 out]
      n81 = Close Reference(reference=w33, error in (no error)=w35) -> ()  [unwired: 1 out]
      n82 = Close Reference(reference=w32, error in (no error)=w30) -> ()  [unwired: 1 out]
      n83 = Close Reference(reference=w27, error in (no error)=w29) -> ()  [unwired: 1 out]
      n84 = Close Reference(reference=w41, error in (no error)=w37) -> ()  [unwired: 1 out]
      n85 = Close Reference(reference=w40, error in (no error)=w38) -> ()  [unwired: 1 out]
      n86 = Close Reference(reference=w44, error in (no error)=w43) -> ()  [unwired: 1 out]
    }
    frame False {
      n87 = Unbundle By Name(w132) -> ("Motion Module.SwaySpeed Set"=w205:refnum<vi>)
      n88 = Unbundle By Name(w132) -> ("Motion Module.Scartch Offset"=w208:refnum<vi>)
      n89 = Unbundle By Name(w132) -> ("Motion Module.Enter Scratch length (mm):"=w211:refnum<vi>)
      n90 = Unbundle By Name(w132) -> ("Motion Module.Enter Scratch Speed (mm/s):"=w200:refnum<vi>)
      n91 = Unbundle By Name(w132) -> ("Motion Module.Motion type:"=w197:refnum<vi>)
      n92 = Unbundle By Name(w132) -> ("Motion Module.Scratch Mode"=w203:refnum<vi>)
      n93 = Unbundle By Name(w132) -> ("Traction reciepe.SRR Sweep Range (%) Stribeck"=w167:refnum<vi>)
      n94 = Unbundle By Name(w132) -> ("Traction reciepe.Traction Receipe"=w170:refnum<vi>)
      n95 = Unbundle By Name(w132) -> ("Traction reciepe.Total Execution Time"=w173:refnum<vi>)
      n96 = Unbundle By Name(w132) -> ("Traction reciepe.Total Steps"=w165:refnum<vi>)
      n97 = Unbundle By Name(w132) -> ("Traction reciepe.Duration / Step (s)  Stribeck"=w162:refnum<vi>)
      n98 = Unbundle By Name(w132) -> ("Traction reciepe.STRIBECK Fixed SRR List (%)"=w159:refnum<vi>)
      n99 = Unbundle By Name(w132) -> ("Traction reciepe.Duration / Step (s) Traction"=w182:refnum<vi>)
      n100 = Unbundle By Name(w132) -> ("Traction reciepe.SRR Sweep Range (%) traction"=w146:refnum<vi>)
      n101 = Unbundle By Name(w132) -> ("Traction reciepe.Rolling Speed (mm/s)"=w143:refnum<vi>)
      n102 = Unbundle By Name(w132) -> ("Traction reciepe.Temperature Stages (°C)"=w140:refnum<vi>)
      n103 = Unbundle By Name(w132) -> ("Traction reciepe.Ball Load (N)"=w148:refnum<vi>)
      n104 = Unbundle By Name(w132) -> ("Traction reciepe.Lubricant Name"=w151:refnum<vi>)
      n105 = Unbundle By Name(w132) -> ("Traction reciepe.Profile File Name"=w154:refnum<vi>)
      n106 = Unbundle By Name(w132) -> ("Motion Module.HomeRot"=w244:refnum<vi>)
      n107 = Unbundle By Name(w132) -> ("Motion Module.HomeScratch"=w239:refnum<vi>)
      n108 = Unbundle By Name(w132) -> ("Motion Module.PlaceModule"=w237:refnum<vi>)
      n109 = Unbundle By Name(w132) -> ("Motion Module.Motion Mode:"=w230:refnum<vi>)
      n110 = Unbundle By Name(w132) -> ("Motion Module.Motion Direction:  3"=w229:refnum<vi>)
      n111 = Unbundle By Name(w132) -> ("Motion Module.Wear Track Diameter (mm)"=w223:refnum<vi>)
      n112 = Unbundle By Name(w132) -> ("Motion Module.Set WTD"=w220:refnum<vi>)
      n113 = Unbundle By Name(w132) -> ("Motion Module.Rotary Module Selection"=w215:refnum<vi>)
      n114 = Unbundle By Name(w132) -> ("Motion Module.No of Scratch"=w186:refnum<vi>)
      n115 = property class="TabCtl (strict)"(reference=w215, "Visible"=FALSE) -> (reference out=w214:refnum<vi>, error out=w216:errorcluster)  [unwired: 1 in]
      n116 = property class="Bool (strict)"(reference=w244, error in=w245, "Visible"=FALSE) -> (reference out=w242:refnum<vi>, error out=w243:errorcluster)
      n117 = property class="Bool (strict)"(reference=w239, error in=w245, "Visible"=FALSE) -> (reference out=w241:refnum<vi>, error out=w240:errorcluster)
      n118 = property class="Bool (strict)"(reference=w237, error in=w245, "Visible"=TRUE) -> (reference out=w235:refnum<vi>, error out=w236:errorcluster)
      n119 = property class="Ring (strict)"(reference=w230, error in=w245, "Visible"=FALSE) -> (reference out=w232:refnum<vi>, error out=w231:errorcluster)
      n120 = property class="Ring (strict)"(reference=w229, error in=w245, "Visible"=FALSE) -> (reference out=w226:refnum<vi>, error out=w228:errorcluster)
      n121 = property class="DigNum (strict)"(reference=w223, "Visible"=FALSE) -> (reference out=w222:refnum<vi>, error out=w224:errorcluster)  [unwired: 1 in]
      n122 = property class="Bool (strict)"(reference=w220, "Visible"=FALSE) -> (reference out=w221:refnum<vi>, error out=w219:errorcluster)  [unwired: 1 in]
      n123 = property class="DigNum (strict)"(reference=w208, "Visible"=FALSE) -> (reference out=w207:refnum<vi>, error out=w209:errorcluster)  [unwired: 1 in]
      n124 = property class="DigNum (strict)"(reference=w211, "Visible"=FALSE) -> (reference out=w212:refnum<vi>, error out=w210:errorcluster)  [unwired: 1 in]
      n125 = property class="DigNum (strict)"(reference=w200, "Visible"=FALSE) -> (reference out=w199:refnum<vi>, error out=w201:errorcluster)  [unwired: 1 in]
      n126 = property class="DigNum (strict)"(reference=w186, "Visible"=FALSE) -> (reference out=w188:refnum<vi>, error out=w187:errorcluster)  [unwired: 1 in]
      n127 = property class="Str"(reference=w167, "Visible"=FALSE) -> (reference out=w168:refnum<vi>, error out=w166:errorcluster)  [unwired: 1 in]
      n128 = property class="MCListbox (strict)"(reference=w170, "Visible"=FALSE) -> (reference out=w169:refnum<vi>, error out=w171:errorcluster)  [unwired: 1 in]
      n129 = property class="DigNum (strict)"(reference=w173, "Visible"=FALSE) -> (reference out=w174:refnum<vi>, error out=w172:errorcluster)  [unwired: 1 in]
      n130 = property class="DigNum (strict)"(reference=w165, "Visible"=FALSE) -> (reference out=w160:refnum<vi>, error out=w164:errorcluster)  [unwired: 1 in]
      n131 = property class="DigNum (strict)"(reference=w162, "Visible"=FALSE) -> (reference out=w161:refnum<vi>, error out=w163:errorcluster)  [unwired: 1 in]
      n132 = property class="Str"(reference=w159, "Visible"=FALSE) -> (reference out=w157:refnum<vi>, error out=w158:errorcluster)  [unwired: 1 in]
      n133 = property class="DigNum (strict)"(reference=w182, "Visible"=FALSE) -> (reference out=w184:refnum<vi>, error out=w183:errorcluster)  [unwired: 1 in]
      n134 = property class="Str"(reference=w146, "Visible"=FALSE) -> (reference out=w145:refnum<vi>, error out=w147:errorcluster)  [unwired: 1 in]
      n135 = property class="DigNum (strict)"(reference=w143, "Visible"=FALSE) -> (reference out=w144:refnum<vi>, error out=w142:errorcluster)  [unwired: 1 in]
      n136 = property class="Str"(reference=w140, "Visible"=FALSE) -> (reference out=w139:refnum<vi>, error out=w141:errorcluster)  [unwired: 1 in]
      n137 = property class="Str"(reference=w148, "Visible"=FALSE) -> (reference out=w153:refnum<vi>, error out=w149:errorcluster)  [unwired: 1 in]
      n138 = property class="Str"(reference=w151, "Visible"=FALSE) -> (reference out=w152:refnum<vi>, error out=w150:errorcluster)  [unwired: 1 in]
      n139 = property class="Str"(reference=w154, "Visible"=FALSE) -> (reference out=w156:refnum<vi>, error out=w155:errorcluster)  [unwired: 1 in]
      n140 = property class="Bool (strict)"(reference=w205, "Visible"=FALSE) -> (reference out=w206:refnum<vi>, error out=w204:errorcluster)  [unwired: 1 in]
      n141 = property class="Ring (strict)"(reference=w203, "Visible"=FALSE) -> (reference out=w198:refnum<vi>, error out=w202:errorcluster)  [unwired: 1 in]
      n142 = property class="Ring (strict)"(reference=w197, "Visible"=FALSE) -> (reference out=w195:refnum<vi>, error out=w196:errorcluster)  [unwired: 1 in]
      n143 = Close Reference(reference=w242, error in (no error)=w243) -> ()  [unwired: 1 out]
      n144 = Close Reference(reference=w241, error in (no error)=w240) -> ()  [unwired: 1 out]
      n145 = Close Reference(reference=w235, error in (no error)=w236) -> ()  [unwired: 1 out]
      n146 = Close Reference(reference=w232, error in (no error)=w231) -> ()  [unwired: 1 out]
      n147 = Close Reference(reference=w226, error in (no error)=w228) -> ()  [unwired: 1 out]
      n148 = Close Reference(reference=w222, error in (no error)=w224) -> ()  [unwired: 1 out]
      n149 = Close Reference(reference=w214, error in (no error)=w216) -> ()  [unwired: 1 out]
      n150 = Close Reference(reference=w221, error in (no error)=w219) -> ()  [unwired: 1 out]
      n151 = Close Reference(reference=w188, error in (no error)=w187) -> ()  [unwired: 1 out]
      n152 = Close Reference(reference=w206, error in (no error)=w204) -> ()  [unwired: 1 out]
      n153 = Close Reference(reference=w207, error in (no error)=w209) -> ()  [unwired: 1 out]
      n154 = Close Reference(reference=w212, error in (no error)=w210) -> ()  [unwired: 1 out]
      n155 = Close Reference(reference=w198, error in (no error)=w202) -> ()  [unwired: 1 out]
      n156 = Close Reference(reference=w199, error in (no error)=w201) -> ()  [unwired: 1 out]
      n157 = Close Reference(reference=w195, error in (no error)=w196) -> ()  [unwired: 1 out]
      n158 = Close Reference(reference=w168, error in (no error)=w166) -> ()  [unwired: 1 out]
      n159 = Close Reference(reference=w169, error in (no error)=w171) -> ()  [unwired: 1 out]
      n160 = Close Reference(reference=w174, error in (no error)=w172) -> ()  [unwired: 1 out]
      n161 = Close Reference(reference=w160, error in (no error)=w164) -> ()  [unwired: 1 out]
      n162 = Close Reference(reference=w161, error in (no error)=w163) -> ()  [unwired: 1 out]
      n163 = Close Reference(reference=w157, error in (no error)=w158) -> ()  [unwired: 1 out]
      n164 = Close Reference(reference=w184, error in (no error)=w183) -> ()  [unwired: 1 out]
      n165 = Close Reference(reference=w145, error in (no error)=w147) -> ()  [unwired: 1 out]
      n166 = Close Reference(reference=w144, error in (no error)=w142) -> ()  [unwired: 1 out]
      n167 = Close Reference(reference=w139, error in (no error)=w141) -> ()  [unwired: 1 out]
      n168 = Close Reference(reference=w153, error in (no error)=w149) -> ()  [unwired: 1 out]
      n169 = Close Reference(reference=w152, error in (no error)=w150) -> ()  [unwired: 1 out]
      n170 = Close Reference(reference=w156, error in (no error)=w155) -> ()  [unwired: 1 out]
    }
  }
  "error out" <- w10
  n171 = Unbundle By Name("Data Cluster") -> ("Main Home Screen.GUI"=w4:refnum<vi>)
  n172 = Unbundle By Name("Data Cluster") -> ("Main Home Screen.MainPage"=w8:refnum<vi>)
  n173 = Unbundle By Name("Data Cluster") -> ("Motion Module.M3 Image"=w11:refnum<vi>)
  n174 = property class="TabCtl (strict)"(reference=w8, "Value"=T2."HOME") -> (reference out=w6:refnum<vi>, error out=w7:errorcluster)  [unwired: 1 in]
  n175 = property class="TabCtl (strict)"(reference=w11, "Value"=enum32{"Page 1", "Page 2"}."Page 2") -> (reference out=w13:refnum<vi>, error out=w12:errorcluster)  [unwired: 1 in]
  n176 = property class="TabCtl (strict)"(reference=w4, "Value"=T3."Motion Module") -> (reference out=w2:refnum<vi>, error out=w3:errorcluster)  [unwired: 1 in]
  n177 = Close Reference(reference=w6, error in (no error)=w7) -> ()  [unwired: 1 out]
  n178 = Close Reference(reference=w13, error in (no error)=w12) -> ()  [unwired: 1 out]
  n179 = Close Reference(reference=w2, error in (no error)=w3) -> ()  [unwired: 1 out]
